vi "Main.vi"(6 "DVR API Suffix":string=" API", 8 "error in (no error)":errorcluster, 9 "DVR API Folder Name":string="APIs", 10 "Method Folder Name":string="Methods", 11 "Class Path":path) -> (0 "error out":errorcluster)   [LabVIEW 2016, in "SLL Scripting.lvlib" / "SLL Class DVR API Generator.lvlib"]
doc: "Generates DVR based APIs for the class methods. \n\nSpecify the \n1. Class path, \n2. Methods folder where the class methods are present,\n3. DVR API folder where the DVR APIs needs to be created,\n4. Suffix for the DVR APIs to be generated"
uses:
  SLL Class DVR API Generator.lvlib
  SLL File IO/SLL File IO.lvlib
panel:
  out "DVR API Count":i32
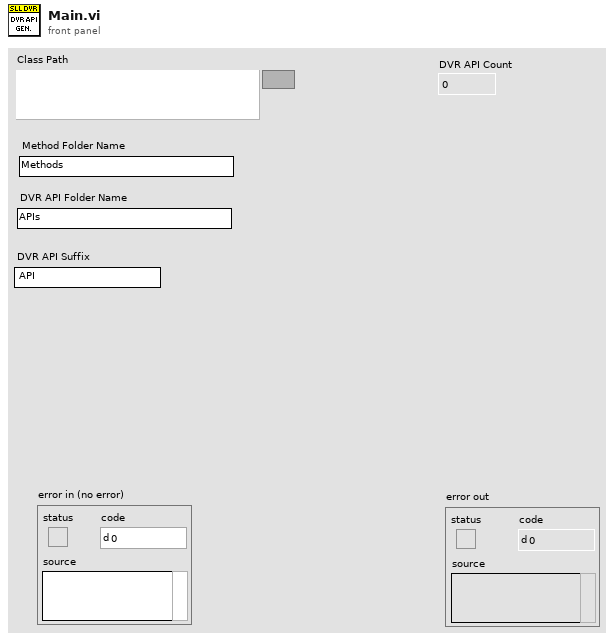
[diagram p1: front panel]
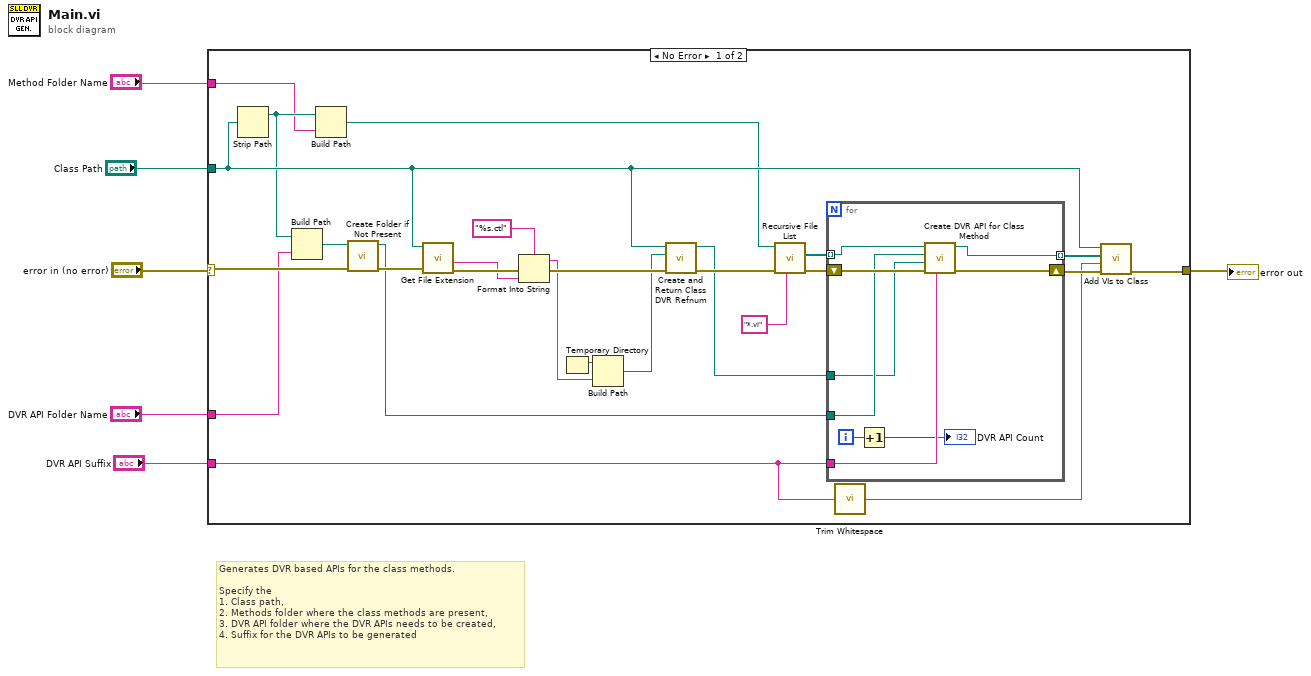
[diagram p0: block diagram]
diagram:
  # "Generates DVR based APIs for the class methods. \n\nSpecify the \n1. Class path, \n2. Methods folder where the class methods are present,\n3. DVR API folder where the DVR APIs needs to be created,\n4. Suffix for the DVR APIs to be generated"
  n1 = case shown="No Error" "error in (no error)" {
    selector: "error in (no error)" -> [w15 w42]
    tunnel: [w19 w42] -> w5
    tunnel: "Class Path" -> [w13 _]
    tunnel: "DVR API Suffix" -> [w18 _]
    tunnel: "DVR API Folder Name" -> [w11 _]
    tunnel: "Method Folder Name" -> [w7 _]
    frame No Error {
      n2 = Strip Path(path=w13) -> (stripped path=w8:path)  [unwired: 1 out]
      n3 = Build Path(base path=w8, name or relative path=w11) -> (appended path=w12:path)
      n4 = Build Path(base path=w8, name or relative path=w7) -> (appended path=w9:path)
      n5 = call "Create Folder if Not Present.vi"("error in (no error)"=w15, "Path"=w12) -> ("error out"=w14:errorcluster, "Path out"=w10:path)  [unwired: 8 in]
      n6 = call <vilib>:"Get File Extension.vi"("error in (no error)"=w14, "file"=w13) -> ("error out"=w28:errorcluster, "filename without extension"=w27:string)  [unwired: 5 in, 3 out]
      n7 = Format Into String(format string="%s.ctl", error in=w28, w27) -> (resulting string=w30:string, error out=w32:errorcluster)  [unwired: 1 in]
      n8 = Temporary Directory() -> (w29:path)
      n9 = Build Path(base path=w29, name or relative path=w30) -> (appended path=w25:path)
      n10 = call "Create and Return Class DVR Refnum.vi"("error in (no error)"=w32, "Path to Save DVR Class Control"=w25, "Class Path"=w13) -> ("error out"=w26:errorcluster, "DVR Class Control Path Out"=w22:path)  [unwired: 7 in]
      n11 = call <vilib>:"Recursive File List.vi"("pattern"="*.vi", "error in (no error)"=w26, "Folder Path"=w9) -> ("error out"=w24:errorcluster, "All Files in Dir"=w21:path[])  [unwired: 4 in, 3 out]
      n12 = for {
        tunnel: w18 -> [w36]
        tunnel: w10 -> [w39]
        tunnel: w22 -> [w38]
        shift-right: [w41] -> w20
        shift-left: w24 -> [w40]
        tunnel: w21 -> [w37] mode=indexing
        tunnel: [w35] -> w16 mode=indexing
        i -> [w34]
        n13 = Increment(x=w34) -> (x+1=→"DVR API Count":i32)
        n14 = call "Create DVR API for Class Method.vi"("DVR API Suffix"=w36, "error in (no error)"=w40, "Class DVR Control File Path"=w38, "DVR API Directory Path"=w39, "Class Method Path"=w37) -> ("error out"=w41:errorcluster, "DVR VI Path"=w35:path)  [unwired: 5 in]
      }
      n15 = call <vilib>:"Trim Whitespace.vi"("string"=w18) -> ("trimmed string"=w17:string)  [unwired: 1 in]
      n16 = call "Add VIs to Class.vi"("error in (no error)"=w20, "Folder Name"=w17, "DVR VI Paths[]"=w16, "Class Path"=w13) -> ("error out"=w19:errorcluster)  [unwired: 7 in]
    }
    frame Error {
    }
  }
  "error out" <- w5
